vi "Configure N5222A.vi"(8 "error in (no error)":errorcluster, 11 "N5222A PNA in":refnum<class "N5222A PNA.lvclass">) -> (0 "error out":errorcluster, 3 "N5222A PNA out":refnum<class "N5222A PNA.lvclass">)   [LabVIEW 2018, in "N5222A PNA.lvclass"]
uses:
  N5222A PNA.lvclass
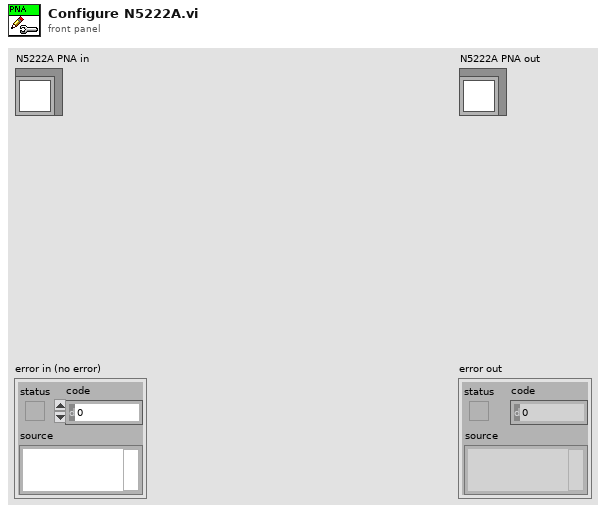
[diagram p1: front panel]
types:
  T1 = typedef "N5222AConfig.ctl" = cluster{"ResourceName":string, "Enable":bool, "Channel":i32, "CalFileName":string, "MeasName":string, "TempDatFile":string, "Power, dBm":dbl, "NumPoints":i32, "Start Freq, Hz":dbl, "Stop Freq, Hz":dbl, "NumAverages":i32, "Sweep Type":i32}
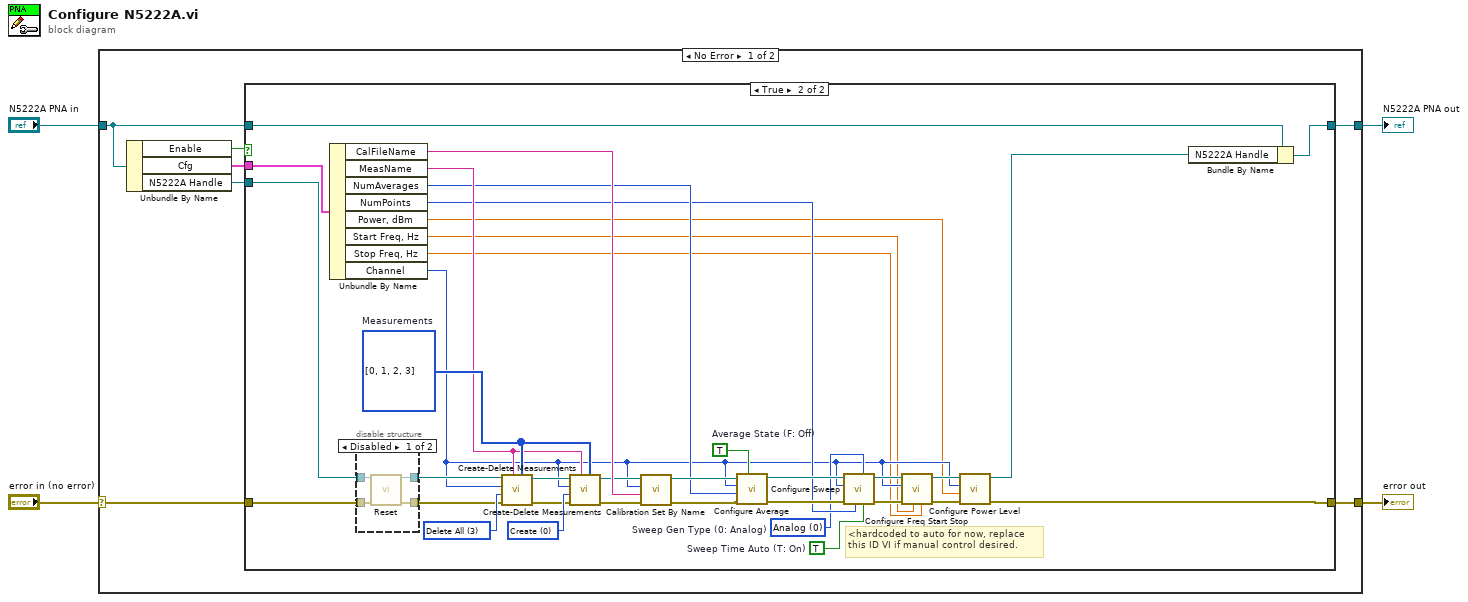
[diagram p0: block diagram]
diagram:
  n1 = case shown="No Error" "error in (no error)" {
    selector: "error in (no error)" -> [w9 w56]
    tunnel: [w8 w56] -> w3
    tunnel: [w6 w55] -> w1
    tunnel: "N5222A PNA in" -> [w7 w55]
    frame No Error {
      n2 = Unbundle By Name(w7) -> ("Enable"=w11:bool, "Cfg"=w10:T1, "N5222A Handle"=w5:refnum<visa-resource-name>)
      n3 = case shown="True" w11 {
        tunnel: w10 -> [_ w48]
        tunnel: [w12 w15] -> w8
        tunnel: w9 -> [w12 w43]
        tunnel: [w13 w36] -> w6
        tunnel: w7 -> [w13 w37]
        tunnel: w5 -> [_ w42]
        frame False {
        }
        frame True {
          w25 = 0 items=["Analog", "Stepped"]  # Sweep Gen Type (0: Analog)
          w24 = TRUE  # Sweep Time Auto (T: On)
          w30 = TRUE  # Average State (F: Off)
          w34 = u16 0 items=["Create", "Delete", "Select", "Delete All"] ("Mode (0: Create)")
          w47 = u16 3 items=["Create", "Delete", "Select", "Delete All"] ("Mode (0: Create)")
          w46 = i32[] [0, 1, 2, 3] items=["S11", "S21", "S12", "S22", "A", "B", "R1", "R2", "A/B", "B/A"]  # Measurements
          # "<hardcoded to auto for now, replace\nthis ID VI if manual control desired."
          n4 = Unbundle By Name(w48) -> ("CalFileName"=w39:string, "MeasName"=w40:string, "NumAverages"=w29:i32, "NumPoints"=w26:i32, "Power, dBm"=w16:dbl, "Start Freq, Hz"=w17:dbl, "Stop Freq, Hz"=w18:dbl, "Channel"=w19:i32)
          n5 = disable-structure shown="Disabled" {
            disable-tunnel: [w52 w53] -> w44
            disable-tunnel: w43 -> [w51 w53]
            disable-tunnel: w42 -> [w50 w54]
            disable-tunnel: [w49 w54] -> w41
            frame Disabled {
              n6 = call <instrlib>:"Reset.vi"("VISA Resource Name"=w50, "error in (no error)"=w51) -> ("VISA Resource Name Out"=w49:refnum<visa-resource-name>, "error out"=w52:errorcluster)  [unwired: 12 in]
            }
            frame Enabled {
            }
          }
          n7 = call "Create-Delete Measurements.vi"("Measurements"=w46, "Measurement Name"=w40, "error out"=w44, "Mode (0: Create)"=w47, "Channel (1)"=w19, "VISA session"=w41) -> ("Error Out"=w33:errorcluster, "VISA Resource Name Out"=w45:refnum<visa-resource-name>)  [unwired: 4 in]
          n8 = call "Create-Delete Measurements.vi"("Measurements"=w46, "Measurement Name"=w40, "error out"=w33, "Mode (0: Create)"=w34, "Channel (1)"=w19, "VISA session"=w45) -> ("Error Out"=w35:errorcluster, "VISA Resource Name Out"=w38:refnum<visa-resource-name>)  [unwired: 4 in]
          n9 = call <instrlib>:"Calibration Set By Name.vi"("Error In (no error)"=w35, "Name"=w39, "Channel (1)"=w19, "VISA Resource Name"=w38) -> ("Error Out"=w32:errorcluster, "VISA Resource Name Out"=w31:refnum<visa-resource-name>)  [unwired: 6 in]
          n10 = call <instrlib>:"Configure Average.vi"("Average State (F: Off)"=w30, "Error In (no error)"=w32, "Average Count (1)"=w29, "Channel (1)"=w19, "VISA Resource Name"=w31) -> ("Error Out"=w28:errorcluster, "VISA Resource Name Out"=w27:refnum<visa-resource-name>)  [unwired: 5 in]
          n11 = call <instrlib>:"Configure Sweep.vi"("Sweep Time Auto (T: On)"=w24, "Sweep Gen Type (0: Analog)"=w25, "Sweep Points (201)"=w26, "Error In (no error)"=w28, "Channel (1)"=w19, "VISA session"=w27) -> ("Error Out"=w22:errorcluster, "dup VISA session"=w23:refnum<visa-resource-name>)  [unwired: 4 in]
          n12 = call <instrlib>:"Configure Freq Start Stop.vi"("Stop Freq (3.0 E+9)"=w18, "Start Freq (300.0 E+3)"=w17, "Error In (no error)"=w22, "Channel (1)"=w19, "VISA session"=w23) -> ("Error Out"=w20:errorcluster, "dup VISA session"=w21:refnum<visa-resource-name>)  [unwired: 5 in]
          n13 = call <instrlib>:"Configure Power Level.vi"("Error In (no error)"=w20, "Power Level (0.0)"=w16, "Channel (1)"=w19, "VISA Resource Name"=w21) -> ("Error Out"=w15:errorcluster, "VISA Resource Name Out"=w14:refnum<visa-resource-name>)  [unwired: 6 in]
          n14 = Bundle By Name(cluster=w37, "N5222A Handle"=w14) -> (w36:refnum<class "N5222A PNA.lvclass">)
        }
      }
    }
    frame Error {
    }
  }
  "error out" <- w3
  "N5222A PNA out" <- w1
